vi "Init.vi"(8 "error in":errorcluster, 11 "statvfs info":T1 {"f_flag" format="%x"; "f_fsid" format="%x"}) -> (0 "error out":errorcluster, 3 "Filesystem Statistics out":refnum<class "Filesystem Statistics.lvclass">)   [LabVIEW 2020, in "NI_SFTP.lvlib" / "Filesystem Statistics.lvclass"]
uses:
  <vilib>/net/SFTP/Filesystem Statistics/Filesystem Statistics.lvclass
  <vilib>/net/SFTP/API/Support/statvfs info.ctl
  <vilib>/net/SFTP/Filesystem Statistics/Filesystem Statistics.lvclass/Filesystem Statistics.ctl
  <vilib>/net/SFTP/NI_SFTP.lvlib
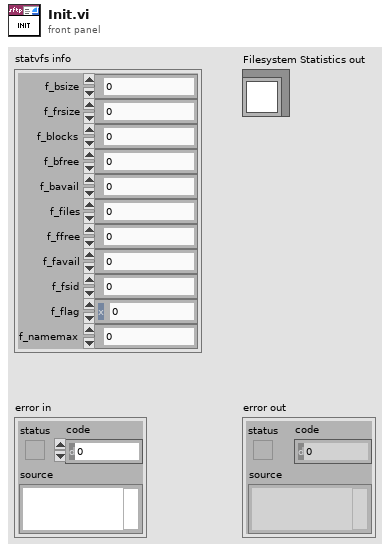
[diagram p1: front panel]
types:
  T1 = typedef "NI_SFTP.lvlib/statvfs info.ctl" = cluster{"f_bsize":u64, "f_frsize":u64, "f_blocks":u64, "f_bfree":u64, "f_bavail":u64, "f_files":u64, "f_ffree":u64, "f_favail":u64, "f_fsid":u64, "f_flag":u64, "f_namemax":u64}
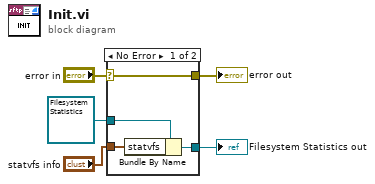
[diagram p0: block diagram]
diagram:
  n1 = case shown="No Error" "error in" {
    selector: "error in" -> [w9 w11]
    tunnel: [w9 w11] -> w4
    tunnel: [w7 w10] -> w2
    tunnel: refnum<class "Filesystem Statistics.lvclass"> refnum ("SFTP Filesystem Statistics in") -> [w6 w10]
    tunnel: "statvfs info" -> [w8 _]
    frame No Error {
      n2 = Bundle By Name(cluster=w6, "statvfs"=w8) -> (w7:refnum<class "Filesystem Statistics.lvclass">)
    }
    frame Error {
    }
  }
  "error out" <- w4
  "Filesystem Statistics out" <- w2
